vi "UHR-Fleezers Control (host) - Lorentz v4.vi"() -> ()   [LabVIEW 2014] (continued)
            n1313 = Subtract(x=w2088, y=w2087) -> (x-y=w2092:dbl)
            n1314 = local write "BD 1 Frequency 2 (MHz)"(w2071) -> ()
            n1315 = Subtract(x=w2082, y=w2071) -> (x-y=w2093:dbl)
            n1316 = Square(x=w2092) -> (x^2=w2090:dbl)
            n1317 = Square(x=w2093) -> (x^2=w2091:dbl)
            n1318 = Add(x=w2091, y=w2090) -> (x+y=w2089:dbl)
            n1319 = Square Root(x=w2089) -> (sqrt(x)=w2086:dbl)
            n1320 = property on="Initial delta (MHz)" class="DigNum (strict)"("Val(Sgnl)"=w2086) -> ()  [unwired: 2 in, 2 out]
            n1321 = local write "Trap Delta (MHz)"(w2086) -> ()
          }
          frame True {
          }
        }
      }
      event "manual raster set": Value Change {
        n1322 = event-data() -> ()  [unwired: 7 out]
        n1323 = flat-sequence {
          frame #0 {
            n1324 = Replace Array Subset(array=u32[] [0] ("Index Values"), new element="manual raster set", index=0) -> (w2113:u32[])
            n1325 = property on="Saved AOD Raster Scan Parameter Sets" class="Arr (strict)"("Index Values"=w2113) -> ()  [unwired: 2 in, 2 out]
          }
          frame #1 {
            n1326 = property on="Load parameters" class="Bool (strict)"("Val(Sgnl)"=TRUE ("Value (Signaling)")) -> ()  [unwired: 2 in, 2 out]
          }
        }
      }
      event "Round T1 X": Value Change {
        n1327 = event-data() -> ()  [unwired: 7 out]
        n1328 = local read "BD 1 Frequency 1 (MHz)"() -> (w2120:dbl)
        n1329 = Round To Nearest(number=w2120) -> (nearest integer value=w2119:dbl)
        n1330 = property on="BD 1 Frequency 1 (MHz)" class="DigNum (strict)"("Val(Sgnl)"=w2119) -> ()  [unwired: 2 in, 2 out]
      }
      event "Round T2 X": Value Change {
        n1331 = event-data() -> ()  [unwired: 7 out]
        n1332 = local read "BD 1 Frequency 2 (MHz)"() -> (w2122:dbl)
        n1333 = Round To Nearest(number=w2122) -> (nearest integer value=w2121:dbl)
        n1334 = property on="BD 1 Frequency 2 (MHz)" class="DigNum (strict)"("Val(Sgnl)"=w2121) -> ()  [unwired: 2 in, 2 out]
      }
      event "Stop All": Value Change {
        n1335 = event-data() -> ()  [unwired: 7 out]
        n1336 = flat-sequence {
          tunnel: [w2128] -> w2126
          tunnel: [w2131] -> w2124
          tunnel: w2126 -> [w2131]
          tunnel: [TRUE] -> w2125
          frame #0 {
            n1337 = local read "Visa resource for valves"() -> (w2127:refnum<visa-resource-name>)
            n1338 = call "hamilton_controller.vi"("VISA resource name in"=w2127, "action"=T53."DISCONNECT") -> ("error out"=w2128:errorcluster)  [unwired: 8 in, 1 out]
          }
          frame #1 {
          }
        }
      }
      event "Delayed Interlace Start": Value Change {
        n1339 = event-data() -> ()  [unwired: 7 out]
        n1340 = flat-sequence {
          frame #0 {
            n1341 = Multiply(x="Delay to Interlace (s)", y=1000.0) -> (x*y=w2133:dbl)
            n1342 = Wait (ms)(milliseconds to wait=w2133) -> ()  [unwired: 1 out]
          }
          frame #1 {
            n1343 = property on="Laser interlacing mode" class="RadioBtnsControl (strict)"("Val(Sgnl)"=enum32{"Laser ON", "Laser OFF", "Interlace"}."Interlace" ("Value (Signaling)")) -> ()  [unwired: 2 in, 2 out]
          }
        }
      }
      event "BD 1 Amplitude 1 (%)", "BD 1 Amplitude 2 (%)", "BD 1 Amplitude 3 (%)", "BD 2 Amplitude 1 (%)", "BD 2 Amplitude 2 (%)", "BD 2 Amplitude 3 (%)", "Trap 1 ON", "Trap 2 ON", "Trap 3 ON", "Feedback On/Off", "All FB On/Off": Value Change {
        w2158 = i16 1 ("f")
        n1344 = event-data() -> ()  [unwired: 7 out]
        n1345 = local write "Trap 1 (ON/OFF)"("Trap 1 ON") -> ()
        n1346 = local write "Trap 2 (ON/OFF)"("Trap 2 ON") -> ()
        n1347 = Boolean To (0,1)(Boolean="Trap 3 ON") -> (0, 1=w2159:i16)
        n1348 = Boolean To (0,1)(Boolean="Trap 1 ON") -> (0, 1=w2160:i16)
        n1349 = Boolean To (0,1)(Boolean="Trap 2 ON") -> (0, 1=w2161:i16)
        n1350 = Select(t=w2161, s="Trap ON/OFF X or Y Amp?", f=w2158) -> (s? t:f=w2156:i16)
        n1351 = Select(t=w2160, s="Trap ON/OFF X or Y Amp?", f=w2158) -> (s? t:f=w2157:i16)
        n1352 = Select(t=w2159, s="Trap ON/OFF X or Y Amp?", f=w2158) -> (s? t:f=w2155:i16)
        n1353 = Select(t=w2158, s="Trap ON/OFF X or Y Amp?", f=w2161) -> (s? t:f=w2153:i16)
        n1354 = Select(t=w2158, s="Trap ON/OFF X or Y Amp?", f=w2160) -> (s? t:f=w2154:i16)
        n1355 = Select(t=w2158, s="Trap ON/OFF X or Y Amp?", f=w2159) -> (s? t:f=w2152:i16)
        n1356 = And(x="All FB On/Off", y="Feedback On/Off") -> (x .and. y?=w2150:cluster{"Set 1":bool, "Set 2":bool})
        n1357 = local read "BD 1 Amplitude 1 (%)"() -> (w2168:dbl)
        n1358 = local read "BD 1 Amplitude 2 (%)"() -> (w2167:dbl)
        n1359 = local read "BD 1 Amplitude 3 (%)"() -> (w2166:dbl)
        n1360 = Unbundle By Name(w2150) -> ("Set 1"=w2145:bool, "Set 2"=w2142:bool)
        n1361 = local read "Y RF Amplitude Limits (%)"() -> (w2138:T24)
        n1362 = local read "X RF Amplitude Limits (%)"() -> (w2139:T24)
        n1363 = local read "BD 2 Amplitude 1 (%)"() -> (w2169:dbl)
        n1364 = local read "BD 2 Amplitude 2 (%)"() -> (w2170:dbl)
        n1365 = local read "BD 2 Amplitude 3 (%)"() -> (w2171:dbl)
        n1366 = And(x="Trap 2 ON", y=w2142) -> (x .and. y?=w2140:bool)
        n1367 = And(x="Trap 1 ON", y=w2145) -> (x .and. y?=w2143:bool)
        n1368 = Multiply(x=w2157, y=w2168) -> (x*y=w2165:dbl)
        n1369 = Multiply(x=w2167, y=w2156) -> (x*y=w2163:dbl)
        n1370 = Multiply(x=w2166, y=w2155) -> (x*y=w2164:dbl)
        n1371 = Multiply(x=w2169, y=w2154) -> (x*y=w2172:dbl)
        n1372 = Multiply(x=w2170, y=w2153) -> (x*y=w2173:dbl)
        n1373 = Multiply(x=w2171, y=w2152) -> (x*y=w2174:dbl)
        n1374 = call "set RF board amplitude - interlace.vi"("Board 2 Amplitude Limits"=w2138, "Board 1 Amplitude Limits"=w2139, "FPGA VI Reference In"=w2137, "Board 2 Amplitude 3 (%)"=w2174, "Board 1 Amplitude 3 (%)"=w2164, "Board 2 Amplitude 2 (%)"=w2173, "Board 2 Amplitude 1 (%)"=w2172, "Board 1 Amplitude 2 (%)"=w2163, "Board 1 Amplitude 1 (%)"=w2165) -> ("error out"=w2147:errorcluster, "FPGA VI Reference Out"=w2148:T50)  [unwired: 1 in]
        n1375 = xnode "Read/Write Control"("FPGA VI Reference In"=w2148, "error in"=w2147, "FB On/Off Set 1"=w2143, "FB On/Off Set 2"=w2140) -> ("error out"=w2146:errorcluster)  [unwired: 1 out]
      }
      event "Load parameters": Value Change {
        n1376 = event-data() -> ()  [unwired: 7 out]
        n1377 = property on="Saved AOD Raster Scan Parameter Sets" class="Arr (strict)"() -> ("Index Values"=w2185:u32[])  [unwired: 2 in, 2 out]
        n1378 = Index Array(array=w2185, index=0) -> (element=w2182:u32)
        n1379 = local write "Load parameters"(FALSE ("Load parameters")) -> ()
        n1380 = Index Array(array="Saved AOD Raster Scan Parameter Sets", index=w2182) -> (element=w2181:T55)
        n1381 = Unbundle By Name(w2181) -> ("Scan Range AOD (nm) 2"=w2180:dbl, "Step Size AOD (nm) 2"=w2179:dbl, "Scan Speed AOD (nm/s) 2"=w2178:dbl, "Number of scans (AOD) 2"=w2177:u16)
        n1382 = flat-sequence {
          tunnel: w2180 -> [w2188]
          tunnel: w2179 -> [w2187]
          tunnel: w2178 -> [w2186]
          tunnel: w2177 -> [w2189]
          frame #0 {
            n1383 = local write "Scan Speed (nm/s)"(w2186) -> ()
            n1384 = local write "Scan Range (nm)"(w2188) -> ()
            n1385 = local write "Step Size (nm)"(w2187) -> ()
          }
          frame #1 {
            n1386 = property on="Number of F/B Scans (AOD)" class="DigNum (strict)"("Val(Sgnl)"=w2189) -> ()  [unwired: 2 in, 2 out]
          }
        }
      }
      event "Trap 1 (ON/OFF)", "Trap 2 (ON/OFF)": Value Change {
        n1387 = event-data() -> ()  [unwired: 7 out]
        n1388 = flat-sequence {
          tunnel: [w2199] -> w2194
          tunnel: w2194 -> [w2214]
          tunnel: [w2200] -> w2190
          frame #0 {
            n1389 = local read "Trap 1 ON"() -> (w2199:bool)
          }
          frame #1 {
            n1390 = Exclusive Or(1:w2214, 2:"Trap 1 (ON/OFF)") -> (0:w2207:bool)
            n1391 = Select(t="on", s="Trap 2 (ON/OFF)", f="off") -> (s? t:f=w2206:string)
            n1392 = Select(t="on", s="Trap 1 (ON/OFF)", f="off") -> (s? t:f=w2202:string)
            n1393 = Build Array("trap 1 ", w2202) -> (w2201:string[])
            n1394 = Build Array("trap 2 " ("f"), w2206) -> (w2204:string[])
            n1395 = Select(t=w2201, s=w2207, f=w2204) -> (s? t:f=w2200:string[])
            n1396 = property on="Trap 1 ON" class="Bool (strict)"("Val(Sgnl)"="Trap 1 (ON/OFF)") -> ()  [unwired: 2 in, 2 out]
            n1397 = property on="Trap 2 ON" class="Bool (strict)"("Val(Sgnl)"="Trap 2 (ON/OFF)") -> ()  [unwired: 2 in, 2 out]
          }
        }
        n1398 = local read "Saving..."() -> (w2193:bool)
        n1399 = local read "Save Event Log?"() -> (w2192:bool)
        n1400 = And(x=w2193, y=w2192) -> (x .and. y?=w2191:bool)
        n1401 = case shown="True" w2191 {
          tunnel: w2190 -> [_ w2198]
          frame False {
          }
          frame True {
            n1402 = local read "Time (s)"() -> (w2195:dbl)
            n1403 = local read "log file ref"() -> (w2197:refnum<file>)
            n1404 = Concatenate Strings(w2198) -> (w2196:string)
            n1405 = call "write to event log.vi"("log file ref"=w2197, "time"=w2195, "input string"=w2196) -> ()  [unwired: 8 in]
          }
        }
      }
      event "DIO count 1 (ticks)", "DIO count 2 (ticks)", "DIO count 3 (ticks)", "Interlace", "Number Interlace Sets", "Not-Interlacing Set", "BD 1 Delay (ticks)", "BD 2 Delay (Ticks)", "Next trap write delay (ticks)", "XY phase ext loop method", "Amp switch delay 2", "BD 2 Delay (Ticks) 2", "BD 1 Delay (ticks) 2": Value Change {
        n1406 = event-data() -> ()  [unwired: 7 out]
        n1407 = To Unsigned Byte Integer(number="Not-Interlacing Set") -> (unsigned 8bit integer=w2215:u8)
        n1408 = Add(x=u8 1 ("y"), y=w2215) -> (x+y=w2224:u8)
        n1409 = local read "DIO count 1 (ticks)"() -> (w2231:u16)
        n1410 = local read "DIO count 2 (ticks)"() -> (w2230:u16)
        n1411 = local read "DIO count 3 (ticks)"() -> (w2229:u16)
        n1412 = xnode "Read/Write Control"("FPGA VI Reference In"=w2217, "DIO count 1 (ticks)"=w2231, "DIO count 2 (ticks)"=w2230, "DIO count 3 (ticks)"=w2229, "Interlace ON/OFF"="Interlace", "Number Interlace Cycles"="Number Interlace Sets", "Interlace Off Parameters"=w2224, "BD 1 Delay (ticks)"="BD 1 Delay (ticks)", "BD 2 Delay (Ticks)"="BD 2 Delay (Ticks)", "Next trap write delay (ticks)"="Next trap write delay (ticks)") -> ("error out"=w2233:errorcluster)  [unwired: 1 in, 1 out]
        n1413 = Build Array(w2231, w2230, w2229) -> (w2223:u16[])
        n1414 = Split 1D Array(array=w2223, index="Number Interlace Sets") -> (first subarray=w2232:u16[])  [unwired: 1 out]
        n1415 = Index Array(array=w2223, index=w2215) -> (element=w2222:u16)
        n1416 = Add Array Elements(numeric array=w2232) -> (sum=w2226:u16)
        n1417 = Select(t=w2226, s="Interlace", f=w2222) -> (s? t:f=→"Total Counts (ticks)":u16)
      }
      event "Reset Feedback": Value Change {
        n1418 = event-data() -> ()  [unwired: 7 out]
        n1419 = Unbundle By Name("Reset Feedback") -> ("Set 1"=w2237:bool, "Set 2"=w2236:bool)
        n1420 = xnode "Read/Write Control"("FPGA VI Reference In"=w2234, "FB Reset Set 1"=w2237, "FB Reset Set 2"=w2236) -> ("error out"=w2235:errorcluster)  [unwired: 1 in, 1 out]
      }
      event "Trap intensity output range", "Trap Intensity PID Gains": Value Change {
        n1421 = event-data() -> ()  [unwired: 7 out]
        n1422 = xnode "Read/Write Control"("FPGA VI Reference In"=w2241, "FB Gains"="Trap Intensity PID Gains", "FB output range"="Trap intensity output range") -> ("error out"=w2242:errorcluster)  [unwired: 1 in, 1 out]
      }
      event "AI2 to Setpoint", "Setpoints (V)": Value Change {
        n1423 = event-data() -> ()  [unwired: 7 out]
        n1424 = xnode "Read/Write Control"("FPGA VI Reference In"=w2243) -> ("FPGA VI Reference Out"=w2246:T50, "error out"=w2245:errorcluster, "AI2 Y Sum Set 1"=w2253:i16, "AI2 Y Sum Set 2"=w2252:i16)  [unwired: 1 in]
        n1425 = Cluster To Array(cluster="AI2 to Setpoint") -> (array=w2256:bool[])
        n1426 = local read "AI2 (V)"() -> (w2254:cluster{"Set 1":dbl, "Set 2":dbl})
        n1427 = Or Array Elements(Boolean array=w2256) -> (logical OR=w2257:bool)
        n1428 = Bundle By Name(cluster=w2254, "Set 1"=w2253, "Set 2"=w2252) -> (w2251:cluster{"Set 1":dbl, "Set 2":dbl})
        n1429 = Divide(x=w2251, y=3276.7) -> (x/y=w2250:cluster{"Set 1":dbl, "Set 2":dbl})
        "AI2 (V)" <- w2250
        n1430 = case shown="True" w2257 {
          tunnel: [w2260 w2277] -> w2249
          tunnel: "AI2 to Setpoint" -> [_ w2273]
          tunnel: "Setpoints (V)" -> [w2261 w2276]
          tunnel: w2250 -> [_ w2270]
          frame False {
            n1431 = Multiply(x=3276.7, y=w2261) -> (x*y=w2262:cluster{"Set 1":dbl, "Set 2":dbl})
            n1432 = To Word Integer(number=w2262) -> (16bit integer=w2260:cluster{"Set 1":i16, "Set 2":i16})
          }
          frame True {
            n1433 = Unbundle By Name(w2270) -> ("Set 1"=w2269:dbl, "Set 2"=w2268:dbl)
            n1434 = Unbundle By Name(w2276) -> ("Set 1"=w2275:dbl, "Set 2"=w2274:dbl)
            n1435 = Unbundle By Name(w2273) -> ("Set 1"=w2272:bool, "Set 2"=w2271:bool)
            n1436 = Select(t=w2269, s=w2272, f=w2275) -> (s? t:f=w2267:dbl)
            n1437 = Select(t=w2268, s=w2271, f=w2274) -> (s? t:f=w2266:dbl)
            n1438 = Bundle By Name(cluster=w2276, "Set 1"=w2267, "Set 2"=w2266) -> (w2264:cluster{"Set 1":dbl, "Set 2":dbl})
            n1439 = local write "Setpoints (V)"(w2264) -> ()
            n1440 = Multiply(x=3276.7, y=w2264) -> (x*y=w2265:cluster{"Set 1":dbl, "Set 2":dbl})
            n1441 = To Word Integer(number=w2265) -> (16bit integer=w2277:cluster{"Set 1":i16, "Set 2":i16})
          }
        }
        n1442 = Unbundle By Name(w2249) -> ("Set 1"=w2248:i16, "Set 2"=w2247:i16)
        n1443 = xnode "Read/Write Control"("FPGA VI Reference In"=w2246, "error in"=w2245, "FB Setpoint Set 1"=w2248, "FB Setpoint Set 2"=w2247) -> ("error out"=w2244:errorcluster)  [unwired: 1 out]
      }
      event "+ phase (GI)", "- phase (GI)", "+ phase (GI) 2", "- phase (GI) 2", "+ phase (RI)", "- phase (RI)", "+ phase (Green FB)", "- phase (Green FB)", "- phase (BI AO)", "+ phase (BI AO)", "- phase (BI DO)", "+ phase (BI DO)": Value Change {
        n1444 = event-data() -> ()  [unwired: 7 out]
        n1445 = Or(x="+ phase (GI)", y="- phase (GI)") -> (x .or. y?=w2313:bool)
        n1446 = Negate(x="Phase adj. (GI)") -> (-x=w2318:i16)
        n1447 = Select(t=w2318, s="+ phase (GI)", f="Phase adj. (GI)") -> (s? t:f=w2317:i16)
        n1448 = Or(x="+ phase (GI) 2", y="- phase (GI) 2") -> (x .or. y?=w2304:bool)
        n1449 = Negate(x="Phase adj. (GI) 2") -> (-x=w2309:i16)
        n1450 = Select(t=w2309, s="+ phase (GI) 2", f="Phase adj. (GI) 2") -> (s? t:f=w2305:i16)
        n1451 = Negate(x="Phase adj. (RI)") -> (-x=w2303:i16)
        n1452 = Or(x="+ phase (RI)", y="- phase (RI)") -> (x .or. y?=w2299:bool)
        n1453 = Select(t=w2303, s="+ phase (RI)", f="Phase adj. (RI)") -> (s? t:f=w2298:i16)
        n1454 = Or(x="+ phase (Green FB)", y="- phase (Green FB)") -> (x .or. y?=w2292:bool)
        n1455 = Negate(x="Phase adj. (Green FB)") -> (-x=w2297:i16)
        n1456 = Select(t=w2297, s="+ phase (Green FB)", f="Phase adj. (Green FB)") -> (s? t:f=w2293:i16)
        n1457 = Negate(x="Phase adj. (BI AO)") -> (-x=w2291:i16)
        n1458 = Or(x="+ phase (BI AO)", y="- phase (BI AO)") -> (x .or. y?=w2281:bool)
        n1459 = Select(t=w2291, s="+ phase (BI AO)", f="Phase adj. (BI AO)") -> (s? t:f=w2283:i16)
        n1460 = Negate(x="Phase adj. (BI DO)") -> (-x=w2287:i16)
        n1461 = Or(x="+ phase (BI DO)", y="- phase (BI DO)") -> (x .or. y?=w2280:bool)
        n1462 = Select(t=w2287, s="+ phase (BI DO)", f="Phase adj. (BI DO)") -> (s? t:f=w2282:i16)
        n1463 = xnode "Read/Write Control"("FPGA VI Reference In"=w2279, "Phase count adjustment (GI)"=w2317, "Phase count adjustment (GI) 2"=w2305, "Phase count adjustment (RI)"=w2298, "Phase count adjustment (Green FB)"=w2293, "Phase count adjustment (BI AO)"=w2283, "Phase count adjustment (BI D)"=w2282) -> ("FPGA VI Reference Out"=w2315:T50, "error out"=w2316:errorcluster)  [unwired: 1 in]
        n1464 = xnode "Read/Write Control"("FPGA VI Reference In"=w2315, "error in"=w2316, "+ phase (GI)"=w2313, "+ phase (GI) 2"=w2304, "+ phase (RI)"=w2299, "+ phase (Green FB)"=w2292, "+ phase (BI AO)"=w2281, "+ phase (BI D)"=w2280) -> ("error out"=w2314:errorcluster)  [unwired: 1 out]
      }
      event "Green Laser ON/OFF", "Red Laser ON/OFF", "Blue Laser ON/OFF": Value Change {
        # "This loop shouldn't be initialized.  The main 'laser ON' settings should dominate and set the others."
        n1465 = event-data() -> ()  [unwired: 7 out]
        n1466 = property on="Red Laser ON" class="Bool (strict)"("Val(Sgnl)"="Red Laser ON/OFF") -> ()  [unwired: 2 in, 2 out]
        n1467 = property on="Blue Laser ON" class="Bool (strict)"("Val(Sgnl)"="Blue Laser ON/OFF") -> ()  [unwired: 2 in, 2 out]
        n1468 = property on="Green Laser ON" class="Bool (strict)"("Val(Sgnl)"="Green Laser ON/OFF") -> ()  [unwired: 2 in, 2 out]
      }
      event "Laser interlacing mode", "Green Laser ON", "Red Laser ON", "Blue Laser ON": Value Change {
        n1469 = event-data() -> ()  [unwired: 7 out]
        n1470 = local write "Green Laser ON/OFF"("Green Laser ON") -> ()
        n1471 = local write "Blue Laser ON/OFF"("Blue Laser ON") -> ()
        n1472 = local write "Red Laser ON/OFF"("Red Laser ON") -> ()
        n1473 = case shown="False" "Green Laser ON" {
          tunnel: "Laser interlacing mode" -> [_ w2379]
          tunnel: [enum32{"Laser ON", "Laser OFF", "Interlace"}."Laser OFF" ("Green laser mode") w2379] -> w2355
          tunnel: [FALSE w2375] -> w2354
          frame False {
          }
          frame True {
            n1474 = local read "Green FB On/Off"() -> (w2376:bool)
            n1475 = Equal?(x=w2379, y=enum32{"Laser ON", "Laser OFF", "Interlace"}."Interlace") -> (x = y?=w2377:bool)
            n1476 = And(x=w2377, y=w2376) -> (x .and. y?=w2375:bool)
          }
        }
        n1477 = case shown="True" "Red Laser ON" {
          tunnel: "Laser interlacing mode" -> [_ w2372]
          tunnel: [enum32{"Laser ON", "Laser OFF", "Interlace"}."Laser OFF" ("Green laser mode") w2372] -> w2351
          tunnel: [FALSE w2368] -> w2350
          frame False {
          }
          frame True {
            n1478 = local read "Red FB On/Off"() -> (w2369:bool)
            n1479 = Equal?(x=w2372, y=enum32{"Laser ON", "Laser OFF", "Interlace"}."Interlace") -> (x = y?=w2370:bool)
            n1480 = And(x=w2370, y=w2369) -> (x .and. y?=w2368:bool)
          }
        }
        n1481 = case shown="True" "Blue Laser ON" {
          tunnel: "Laser interlacing mode" -> [_ w2363]
          tunnel: [enum32{"Laser ON", "Laser OFF", "Interlace"}."Laser OFF" ("Green laser mode") w2363] -> w2347
          tunnel: [FALSE w2361] -> w2346
          frame False {
          }
          frame True {
            n1482 = local read "Blue FB On/Off"() -> (w2362:bool)
            n1483 = Equal?(x=w2363, y=enum32{"Laser ON", "Laser OFF", "Interlace"}."Interlace") -> (x = y?=w2364:bool)
            n1484 = And(x=w2364, y=w2362) -> (x .and. y?=w2361:bool)
          }
        }
        n1485 = xnode "Read/Write Control"("FPGA VI Reference In"=w2345, "Operating Mode"=w2355, "Operating Mode 2"=w2355, "Green FB On/Off"=w2354, "Red Laser Operating Mode"=w2351, "RI Operating Mode 2"=w2351, "Red FB On/Off"=w2350, "BI Operating Mode (AO)"=w2347, "Blue Laser Operating Mode (D)"=w2347, "Blue FB On/Off"=w2346) -> ("error out"=w2356:errorcluster)  [unwired: 1 in, 1 out]
        n1486 = local read "Red FB On/Off"() -> (w2328:bool)
        n1487 = local read "Green FB On/Off"() -> (w2330:bool)
        n1488 = local read "Green Laser ON"() -> (w2329:bool)
        n1489 = local read "Red Laser ON"() -> (w2327:bool)
        n1490 = And(x=w2328, y=w2327) -> (x .and. y?=w2333:bool)
        n1491 = And(x=w2330, y=w2329) -> (x .and. y?=w2339:bool)
        n1492 = local read "Red laser intensity (V)"() -> (w2332:dbl)
        n1493 = local read "Red FB Setpoint (mV)"() -> (w2331:dbl)
        n1494 = local read "Green FB Setpoint (mV)"() -> (w2342:dbl)
        n1495 = local read "Green laser intensity (V)"() -> (w2344:dbl)
        n1496 = Multiply(x=w2332, y=1000.0) -> (x*y=w2336:dbl)
        n1497 = Subtract(x=w2331, y=5.0) -> (x-y=w2335:dbl)
        n1498 = Multiply(x=w2344, y=1000.0) -> (x*y=w2341:dbl)
        n1499 = Subtract(x=w2342, y=5.0) -> (x-y=w2340:dbl)
        n1500 = Less Or Equal?(x=w2336, y=w2335) -> (x <= y?=w2334:bool)
        n1501 = Less Or Equal?(x=w2341, y=w2340) -> (x <= y?=w2338:bool)
        n1502 = And(x=w2333, y=w2334) -> (x .and. y?=w2323:bool)
        n1503 = And(x=w2339, y=w2338) -> (x .and. y?=w2324:bool)
        n1504 = Or(x=w2324, y=w2323) -> (x .or. y?=w2322:bool)
        n1505 = case shown="True" w2322 {
          frame False {
            n1506 = local write "Laser Intensity Low (bugs to fix)"(FALSE ("Laser Intensity Low")) -> ()
          }
          frame True {
            n1507 = local write "Laser Intensity Low (bugs to fix)"(TRUE ("Laser Intensity Low")) -> ()
          }
        }
      }
      event "Invert laser interlacing": Value Change {
        n1508 = event-data() -> ()  [unwired: 7 out]
        n1509 = xnode "Read/Write Control"("FPGA VI Reference In"=w2380, "Invert GI"="Invert laser interlacing", "Invert GI 2"="Invert laser interlacing", "Invert RI"="Invert laser interlacing", "Invert RI 2"="Invert laser interlacing", "Invert BI (AO)"="Invert laser interlacing", "Invert BI (D)"="Invert laser interlacing") -> ("error out"=w2382:errorcluster)  [unwired: 1 in, 1 out]
      }
      event "Green FB Setpoint (mV)", "Green FB Gains", "Green FB On/Off", "Green Intensity % (FB OFF)", "Green int current ON count adj": Value Change {
        n1510 = event-data() -> ()  [unwired: 7 out]
        n1511 = local read "Green FB Setpoint (mV)"() -> (w2402:dbl)
        n1512 = Multiply(x=w2402, y=3.2767) -> (x*y=w2401:dbl)
        n1513 = local read "Green Intensity % (FB OFF)"() -> (w2405:dbl)
        n1514 = Multiply(x=w2405, y=655.35) -> (x*y=w2406:dbl)
        n1515 = To Unsigned Word Integer(number=w2406) -> (unsigned 16bit integer=w2404:u16)
        n1516 = local read "Green int current ON count adj"() -> (w2408:u32)
        n1517 = local read "Laser interlacing mode"() -> (w2399:enum32{"Laser ON", "Laser OFF", "Interlace"})
        n1518 = local read "Green FB Gains"() -> (w2396:T14)
        n1519 = local read "Green Laser ON"() -> (w2400:bool)
        n1520 = local read "Green FB On/Off"() -> (w2409:bool)
        n1521 = Equal?(x=w2399, y=enum32{"Laser ON", "Laser OFF", "Interlace"}."Interlace") -> (x = y?=w2397:bool)
        n1522 = Unbundle By Name(w2396) -> ("proportional gain (Kc)"=w2395:i16, "integral gain (Kc*Ts/Ti)"=w2394:i16, "derivative gain (Kc*Td/Ts)"=w2393:i16)
        n1523 = Compound Arithmetic op=AND(w2397, w2409, w2400) -> (w2383:bool)
        n1524 = local read "Green FB Setpoint (mV)"() -> (w2387:dbl)
        n1525 = local read "Green laser intensity (V)"() -> (w2390:dbl)
        n1526 = xnode "Read/Write Control"("FPGA VI Reference In"=w2392, "Green FB Setpoint"=w2401, "Green FB On/Off"=w2383, "Current Out"=w2404, "Green int current ON count adj"=w2408, "P3"=w2395, "I3"=w2394, "D3"=w2393) -> ("error out"=w2410:errorcluster)  [unwired: 1 in, 1 out]
        n1527 = Multiply(x=w2390, y=1000.0) -> (x*y=w2386:dbl)
        n1528 = Subtract(x=w2387, y=5.0) -> (x-y=w2385:dbl)
        n1529 = Less Or Equal?(x=w2386, y=w2385) -> (x <= y?=w2384:bool)
        n1530 = And(x=w2383, y=w2384) -> (x .and. y?=w2391:bool)
        n1531 = case shown="True" w2391 {
          frame False {
            n1532 = local write "Laser Intensity Low (bugs to fix)"(FALSE ("Laser Intensity Low")) -> ()
          }
          frame True {
            n1533 = local write "Laser Intensity Low (bugs to fix)"(TRUE ("Laser Intensity Low")) -> ()
          }
        }
      }
      event "Blue FB Setpoint (mV)", "Blue FB Gains", "Blue FB On/Off", "Blue Intensity % (FB OFF)", "Blue int AO ON count adjust": Value Change {
        # "Triggers blue laser serial command"
        # "16 bit analog out"
        n1534 = event-data() -> ()  [unwired: 7 out]
        n1535 = Multiply(x="Blue FB Setpoint (mV)", y=3.2767) -> (x*y=w2430:dbl)
        n1536 = Multiply(x="Blue Intensity % (FB OFF)", y=0.8) -> (x*y=w2413:dbl)
        n1537 = Number To Decimal String(number=w2413) -> (decimal integer string=w2414:string)  [unwired: 1 in]
        n1538 = Multiply(x="Blue Intensity % (FB OFF)", y=655.35) -> (x*y=w2433:dbl)
        n1539 = local write "Blue Laser Power (mW)\n(Constant Power Mode)"(w2414) -> ()
        n1540 = To Unsigned Word Integer(number=w2433) -> (unsigned 16bit integer=w2432:u16)
        n1541 = local read "Laser interlacing mode"() -> (w2428:enum32{"Laser ON", "Laser OFF", "Interlace"})
        n1542 = Unbundle By Name("Blue FB Gains") -> ("proportional gain (Kc)"=w2425:i16, "integral gain (Kc*Ts/Ti)"=w2424:i16, "derivative gain (Kc*Td/Ts)"=w2423:i16)
        n1543 = local read "Blue Laser ON"() -> (w2418:bool)
        n1544 = Equal?(x=w2428, y=enum32{"Laser ON", "Laser OFF", "Interlace"}."Interlace") -> (x = y?=w2426:bool)
        n1545 = Compound Arithmetic op=AND(w2426, "Blue FB On/Off", w2418) -> (w2429:bool)
        n1546 = xnode "Read/Write Control"("FPGA VI Reference In"=w2417, "Blue FB Setpoint"=w2430, "Blue FB On/Off"=w2429, "BI Current Out"=w2432, "Blue current ON count adj (AO)"="Blue int AO ON count adjust", "P5"=w2425, "I5"=w2424, "D5"=w2423) -> ("error out"=w2435:errorcluster)  [unwired: 1 in, 1 out]
      }
      event "Red FB Setpoint (mV)", "Red FB Gains", "Red FB On/Off", "Red Intensity % (FB OFF)": Value Change {
        n1547 = event-data() -> ()  [unwired: 7 out]
        n1548 = local read "Red FB Setpoint (mV)"() -> (w2456:dbl)
        n1549 = Multiply(x=w2456, y=3.2767) -> (x*y=w2455:dbl)
        n1550 = local read "Red Intensity % (FB OFF)"() -> (w2446:dbl)
        n1551 = Multiply(x=w2446, y=655.35) -> (x*y=w2459:dbl)
        n1552 = To Unsigned Word Integer(number=w2459) -> (unsigned 16bit integer=w2458:u16)
        n1553 = local read "Laser interlacing mode"() -> (w2453:enum32{"Laser ON", "Laser OFF", "Interlace"})
        n1554 = local read "Red FB Gains"() -> (w2450:T14)
        n1555 = local read "Red Laser ON"() -> (w2454:bool)
        n1556 = local read "Red FB On/Off"() -> (w2461:bool)
        n1557 = Equal?(x=w2453, y=enum32{"Laser ON", "Laser OFF", "Interlace"}."Interlace") -> (x = y?=w2451:bool)
        n1558 = Unbundle By Name(w2450) -> ("proportional gain (Kc)"=w2449:i16, "integral gain (Kc*Ts/Ti)"=w2448:i16, "derivative gain (Kc*Td/Ts)"=w2447:i16)
        n1559 = Compound Arithmetic op=AND(w2451, w2461, w2454) -> (w2438:bool)
        n1560 = local read "Red laser intensity (V)"() -> (w2437:dbl)
        n1561 = local read "Red FB Setpoint (mV)"() -> (w2436:dbl)
        n1562 = xnode "Read/Write Control"("FPGA VI Reference In"=w2445, "Red FB Setpoint"=w2455, "Red FB On/Off"=w2438, "RI Current Out"=w2458, "P4"=w2449, "I4"=w2448, "D4"=w2447) -> ("error out"=w2462:errorcluster)  [unwired: 1 in, 1 out]
        n1563 = Multiply(x=w2437, y=1000.0) -> (x*y=w2442:dbl)
        n1564 = Subtract(x=w2436, y=5.0) -> (x-y=w2441:dbl)
        n1565 = Less Or Equal?(x=w2442, y=w2441) -> (x <= y?=w2440:bool)
        n1566 = And(x=w2438, y=w2440) -> (x .and. y?=w2439:bool)
        n1567 = case shown="False" w2439 {
          frame False {
            n1568 = local write "Laser Intensity Low (bugs to fix)"(FALSE ("Laser Intensity Low")) -> ()
          }
          frame True {
            n1569 = local write "Laser Intensity Low (bugs to fix)"(TRUE ("Laser Intensity Low")) -> ()
          }
        }
      }
      event "+ phase (APD 1 Gate)", "- phase (APD 1 Gate)", "+ phase (APD 2 Gate)", "- phase (APD 2 Gate)", "+ phase (APD 3 Gate)", "- phase (APD 3 Gate)", "+ phase (APD Acq)", "- phase (APD Acq)": Value Change {
        n1570 = event-data() -> ()  [unwired: 7 out]
        n1571 = local read "Phase Adj. (APD 1 Gate)"() -> (w2485:i16)
        n1572 = Or(x="- phase (APD 1 Gate)", y="+ phase (APD 1 Gate)") -> (x .or. y?=w2487:bool)
        n1573 = Negate(x=w2485) -> (-x=w2492:i16)
        n1574 = Select(t=w2492, s="+ phase (APD 1 Gate)", f=w2485) -> (s? t:f=w2491:i16)
        n1575 = local read "Phase Adj. (APD 2 Gate)"() -> (w2482:i16)
        n1576 = Or(x="- phase (APD 2 Gate)", y="+ phase (APD 2 Gate)") -> (x .or. y?=w2480:bool)
        n1577 = Negate(x=w2482) -> (-x=w2484:i16)
        n1578 = Select(t=w2484, s="+ phase (APD 2 Gate)", f=w2482) -> (s? t:f=w2481:i16)
        n1579 = Negate(x="Phase Adj. (APD 3 Gate)") -> (-x=w2479:i16)
        n1580 = Or(x="- phase (APD 3 Gate)", y="+ phase (APD 3 Gate)") -> (x .or. y?=w2475:bool)
        n1581 = Select(t=w2479, s="+ phase (APD 3 Gate)", f="Phase Adj. (APD 3 Gate)") -> (s? t:f=w2476:i16)
        n1582 = local read "Phase Adj. (APD Acq)"() -> (w2473:i16)
        n1583 = Or(x="- phase (APD Acq)", y="+ phase (APD Acq)") -> (x .or. y?=w2471:bool)
        n1584 = Negate(x=w2473) -> (-x=w2474:i16)
        n1585 = Select(t=w2474, s="+ phase (APD Acq)", f=w2473) -> (s? t:f=w2472:i16)
        n1586 = xnode "Read/Write Control"("FPGA VI Reference In"=w2465, "Phase count adjustment (APD 1 Gate)"=w2491, "Phase count adjustment (APD 2 Gate)"=w2481, "Phase count adjustment (APD 3 Gate)"=w2476, "Phase Count Adjustment (APD Acq)"=w2472) -> ("FPGA VI Reference Out"=w2489:T50, "error out"=w2490:errorcluster)  [unwired: 1 in]
        n1587 = xnode "Read/Write Control"("FPGA VI Reference In"=w2489, "error in"=w2490, "+ phase (APD 1 Gate)"=w2487, "+ phase (APD 2 Gate)"=w2480, "+ phase (APD 3 Gate)"=w2475, "+ phase (APD Acq)"=w2471) -> ("error out"=w2488:errorcluster)  [unwired: 1 out]
      }
      event "Invert APD Gate", "APD Gate ON Count", "APD Gate OFF Count", "APD Gate", "APD Integration Time (s)", "APD AO Scale Factor", "Duty Frequency (ON 1/N cycles)", "Interlace ON count", "Interlace OFF count": Value Change {
        n1588 = event-data() -> ()  [unwired: 7 out]
        n1589 = Add(x="Interlace ON count", y="Interlace OFF count") -> (x+y=w2499:u16)
        n1590 = Add(x="APD Gate ON Count", y="APD Gate OFF Count") -> (x+y=w2510:u16)
        n1591 = Multiply(x="Duty Frequency (ON 1/N cycles)", y=w2499) -> (x*y=w2495:u16)
        "Green AI Count" <- w2495
        "Red AI Count" <- w2495
        "Blue AI Count" <- w2495
        n1592 = Subtract(x=w2495, y="Interlace ON count") -> (x-y=w2498:u16)
        n1593 = Multiply(x=w2510, y="Duty Frequency (ON 1/N cycles)") -> (x*y=w2509:u16)
        n1594 = Subtract(x=w2509, y="APD Gate ON Count") -> (x-y=w2508:u16)
        n1595 = local read "DMA Update Period (s)"() -> (w2511:dbl)
        n1596 = Multiply(x="APD Integration Time (s)", y=40000000.0) -> (x*y=w2515:dbl)
        n1597 = Reciprocal(x="APD Integration Time (s)") -> (1/x=→"APD Acq Rate (Hz)":dbl)
        n1598 = To Unsigned Long Integer(number=w2515) -> (unsigned 32bit integer=w2501:u32)
        "APD Int. Count" <- w2501
        n1599 = local read "Number of APDs"() -> (w2494:u8)
        n1600 = Divide(x=w2511, y="APD Integration Time (s)") -> (x/y=w2513:dbl)
        n1601 = Multiply(x=w2494, y=w2513) -> (x*y=w2512:dbl)
        n1602 = local write "APD Samples/FIFO Acq."(w2513) -> ()
        n1603 = local write "APD Elements/DMA read"(w2512) -> ()
        n1604 = xnode "Read/Write Control"("FPGA VI Reference In"=w2493, "Invert APD Gate"="Invert APD Gate", "APD Gate ON Count"="APD Gate ON Count", "APD Gate OFF Count"=w2508, "APD Acq Rate Count"=w2501, "APD Gate Operating Mode"="APD Gate", "APD AO scale factor"="APD AO Scale Factor", "Green interlace ON count"="Interlace ON count", "Green interlace OFF count"=w2498, "Green interlace ON count 2"="Interlace ON count", "Green interlace OFF count 2"=w2498, "Green FB Count"=w2495, "Red interlace ON count"="Interlace ON count", "Red interlace OFF count"="Interlace OFF count", "Blue ON count (AO)"="Interlace ON count", "Blue OFF count (AO)"="Interlace OFF count", "Blue interlace OFF count (D)"="Interlace OFF count", "Blue interlace ON count (D)"="Interlace ON count") -> ("error out"=w2517:errorcluster)  [unwired: 1 in, 1 out]
      }
      event "Neg. TTrig FPGA": Value Change {
        n1605 = event-data() -> ()  [unwired: 7 out]
        n1606 = xnode "Read/Write Control"("FPGA VI Reference In"=w2518, "TTrig Negate Pos"="Neg. TTrig FPGA") -> ()  [unwired: 1 in, 2 out]
      }
      event "Test ttrig": Value Change {
        n1607 = event-data() -> ()  [unwired: 7 out]
        n1608 = xnode "Read/Write Control"("FPGA VI Reference In"=w2520, "TTrig?"=TRUE) -> ("error out"=w2522:errorcluster)  [unwired: 1 in, 1 out]
      }
      event "Number of F/B Scans (AOD)", "Scan Speed (nm/s)", "Scan BD", "Initial delta (MHz)", "Step Size (nm)", "Scan Range (nm)": Value Change {
        w2586 = 123.0  # AOM cal (nm/MHz)
        n1609 = event-data() -> ()  [unwired: 7 out]
        n1610 = local read "BD 1 Frequency 1 (MHz)"() -> (w2569:dbl)
        n1611 = local read "AOM X Cal (nm/MHz)"() -> (w2561:dbl)
        n1612 = local read "X RF Frequency Limits (MHz)"() -> (w2573:T24)
        n1613 = local read "Y RF Frequency Limits (MHz)"() -> (w2570:T24)
        n1614 = local read "BD 2 Frequency 1 (MHz)"() -> (w2575:dbl)
        n1615 = Negate(x="Scan Range (nm)") -> (-x=w2539:dbl)
        n1616 = Divide(x=w2539, y=w2561) -> (x/y=w2543:dbl)
        n1617 = Select(t=w2573, s="Scan BD", f=w2570) -> (s? t:f=w2572:T24)
        n1618 = Select(t=w2569, s="Scan BD", f=w2575) -> (s? t:f=w2574:dbl)
        n1619 = Unbundle By Name(w2572) -> ("Maximum"=w2581:dbl, "Minimum"=w2580:dbl)
        n1620 = Add(x=w2543, y=w2574) -> (x+y=w2578:dbl)
        n1621 = Divide(x=w2539, y="Step Size (nm)") -> (x/y=w2558:dbl)
        n1622 = Divide(x="Step Size (nm)", y=w2561) -> (x/y=w2567:dbl)
        n1623 = Absolute Value(x=w2558) -> (abs(x)=w2542:dbl)
        n1624 = Sign(1:w2539) -> (0:w2540:dbl)
        n1625 = In Range and Coerce(upper limit=w2581, x=w2578, lower limit=w2580) -> (coerced(x)=w2577:dbl, In Range?=w2579:bool)
        n1626 = To Unsigned Quad Integer(1:w2542) -> (0:w2557:u64)
        "Scan steps (AOD)" <- w2557
        n1627 = call "IR AOM freq to word.vi"("Frequency In (MHz)"=w2567) -> ("Frequency Word Out (double)"=w2564:dbl)
        n1628 = Multiply(x=w2540, y=w2564) -> (x*y=w2541:dbl)
        n1629 = Subtract(x=w2578, y=w2577) -> (x-y=w2576:dbl)
        n1630 = To Quad Integer(1:w2541) -> (0:w2563:i64)
        "Incr. int (AOD)" <- w2563
        n1631 = Subtract(x=w2543, y=w2576) -> (x-y=w2562:dbl)
        "Scan Range (MHz)" <- w2562
        n1632 = Select(t=w2543, s=w2579, f=w2562) -> (s? t:f=w2582:dbl)
        n1633 = Multiply(x=w2562, y=w2561) -> (x*y=w2560:dbl)
        n1634 = Decrement(x=w2557) -> (x-1=w2610:u64)
        n1635 = Negate(x=w2560) -> (-x=w2556:dbl)
        n1636 = local write "Scan Range (nm)"(w2556) -> ()
        n1637 = Divide(x=w2582, y=w2610) -> (x/y=w2566:dbl)
        "Scan Increment (MHz)" <- w2566
        n1638 = call "IR AOM freq to word.vi"("Frequency In (MHz)"=w2566) -> ("Frequency Word Out (double)"=w2565:dbl)
        n1639 = Divide(x="Step Size (nm)", y="Scan Speed (nm/s)") -> (x/y=w2553:dbl)
        n1640 = To Quad Integer(1:w2565) -> ()  [unwired: 1 out]
        n1641 = local read "Number Interlace Sets"() -> (w2537:u8)
        n1642 = local read "AI Count (ticks)"() -> (w2538:u16)
        n1643 = local read "Total Counts (ticks)"() -> (w2536:u16)
        n1644 = local read "# Samples/trap"() -> (w2568:u32)
        n1645 = Multiply(x=w2538, y=w2537) -> (x*y=w2535:u16)
        n1646 = Divide(x=w2536, y=w2535) -> (x/y=w2534:dbl)
        n1647 = Select(t=w2569, s="Scan BD", f=w2575) -> (s? t:f=w2607:dbl)
        "Initial freq. (MHz)" <- w2607
        n1648 = Add(x=w2582, y=w2607) -> (x+y=→"Final freq. (MHz)":dbl)
        n1649 = Divide(x=w2536, y=40000000.0) -> (x/y=w2552:dbl)
        n1650 = Divide(x=w2553, y=w2552) -> (x/y=w2551:dbl)
        n1651 = To Unsigned Quad Integer(1:w2551) -> (0:w2526:u64)
        n1652 = Quotient & Remainder(x=w2526, y=u64 2) -> (x-y*floor(x/y)=w2530:u64)  [unwired: 1 out]
        n1653 = Equal?(x=w2530, y=u64 0) -> (x = y?=w2528:bool)
        n1654 = Decrement(x=w2526) -> (x-1=w2527:u64)
        n1655 = Select(t=w2526, s=w2528, f=w2527) -> (s? t:f=w2525:u64)
        "Cycles/step (AOD)" <- w2525
        n1656 = xnode "Read/Write Control"("FPGA VI Reference In"=w2524, "Scan steps"=w2557, "Number of scans"="Number of F/B Scans (AOD)", "Cycles per step"=w2525, "Scan freq.  increment"=w2563, "Scan BD"="Scan BD") -> ("error out"=w2616:errorcluster)  [unwired: 1 in, 1 out]
        n1657 = Multiply(x=w2557, y=w2525) -> (x*y=w2611:u64)
        n1658 = Multiply(x=w2611, y=u64 2) -> (x*y=w2533:u64)
        n1659 = Multiply(x=w2534, y=w2533) -> (x*y=w2532:dbl)
        "Data points/scan (f/b)" <- w2532
        n1660 = Multiply(x=w2532, y="Number of F/B Scans (AOD)") -> (x*y=w2614:dbl)
        "Data points/scans" <- w2614
        n1661 = Divide(x=w2614, y=w2568) -> (x/y=→"N sets should be saved":dbl)
        n1662 = Multiply(x=w2611, y=w2552) -> (x*y=w2550:dbl)
        "Time/Scan (s) (AOD)" <- w2550
        n1663 = Select(t=w2582, s="Scan BD", f=0.0) -> (s? t:f=w2608:dbl)
        n1664 = Select(t=0.0, s="Scan BD", f=w2582) -> (s? t:f=w2604:dbl)
        n1665 = local read "BD 2 Frequency 2 (MHz)"() -> (w2600:dbl)
        n1666 = local read "BD 1 Frequency 2 (MHz)"() -> (w2603:dbl)
        n1667 = Add(x=w2604, y=w2575) -> (x+y=w2601:dbl)
        n1668 = Add(x=w2569, y=w2608) -> (x+y=w2602:dbl)
        n1669 = Multiply(x=w2550, y=2.0) -> (x*y=w2549:dbl)
        n1670 = Multiply(x=w2549, y="Number of F/B Scans (AOD)") -> (x*y=w2546:dbl)
        n1671 = Divide(x=w2546, y=60.0) -> (x/y=→"Time to Finish All (min)":dbl)
        n1672 = Add(x="Trap 2 Bead Size (nm)", y="Trap 1 Bead Size (nm)") -> (x+y=w2590:dbl)
        n1673 = Divide(x=w2590, y=2.0) -> (x/y=w2584:dbl)
        n1674 = local read "Initial delta (MHz)"() -> (w2587:dbl)
        n1675 = Subtract(x=w2601, y=w2600) -> (x-y=w2598:dbl)
        n1676 = Subtract(x=w2602, y=w2603) -> (x-y=w2599:dbl)
        n1677 = Square(x=w2598) -> (x^2=w2597:dbl)
        n1678 = Square(x=w2599) -> (x^2=w2596:dbl)
        n1679 = Add(x=w2596, y=w2597) -> (x+y=w2595:dbl)
        n1680 = Square Root(x=w2595) -> (sqrt(x)=w2594:dbl)
        "Final delta (MHz)" <- w2594
        n1681 = Multiply(x=w2586, y=w2594) -> (x*y=w2593:dbl)
        n1682 = Multiply(x=w2587, y=w2586) -> (x*y=w2585:dbl)
        n1683 = Subtract(x=w2585, y=w2584) -> (x-y=→"Initial sep (nm)":dbl)
        n1684 = Subtract(x=w2593, y=w2584) -> (x-y=→"Final sep (nm)":dbl)
      }
      event "Freq or Amp switch first", "Swap F1 and F2", "Freq switch delay", "Amp switch delay": Value Change {
        n1685 = event-data() -> ()  [unwired: 7 out]
        n1686 = local read "Amp switch delay"() -> (w2618:u16)
        n1687 = local read "Swap F1 and F2"() -> (w2619:bool)
        n1688 = xnode "Read/Write Control"("FPGA VI Reference In"=w2617, "Swap F1 and F2"=w2619, "Amp switch delay"=w2618) -> ("error out"=w2620:errorcluster)  [unwired: 1 in, 1 out]
      }
      event "Scan steps (MCL)", "Number of scans (MCL)", "Scan Range (V)\n(of steps)", "2D or 1D Scan", "N APD Samp/step", "Fast Scan Dir", "Continuous MCL Scanning", "Scan lines (y)": Value Change {
        w2623 = 32767.0 ("y")
        n1689 = event-data() -> ()  [unwired: 7 out]
        n1690 = Select(t="Scan lines (y)", s="2D or 1D Scan", f="Number of scans (MCL)") -> (s? t:f=w2628:u64)
        n1691 = Decrement(x="Scan steps (MCL)") -> (x-1=w2644:u64)
        n1692 = Divide(x="Scan Range (V)\n(of steps)", y=w2644) -> (x/y=w2643:dbl)
        "Desired Scan Incr (V)" <- w2643
        n1693 = local read "APD Integration Time (s)"() -> (w2636:dbl)
        n1694 = Multiply(x=w2643, y=w2623) -> (x*y=w2652:dbl)
        n1695 = Divide(x=w2652, y=10.0) -> (x/y=w2642:dbl)
        "Desired incr (int)" <- w2642
        n1696 = local read "Update Count (MCL)"() -> (w2648:u32)
        n1697 = Round Toward -Infinity(1:w2642) -> (0:w2651:dbl)
        n1698 = To Word Integer(number=w2651) -> (16bit integer=w2626:i16)
        "Actual Incr. int (MCL)" <- w2626
        n1699 = Multiply(x=w2636, y=40000000.0) -> (x*y=w2649:dbl)
        n1700 = Divide(x=w2649, y=w2648) -> (x/y=w2647:dbl)
        n1701 = Multiply(x=i16 10, y=w2626) -> (x*y=w2624:i16)
        n1702 = Multiply(x="N APD Samp/step", y=w2647) -> (x*y=w2646:dbl)
        "Cycles/step (MCL)" <- w2646
        n1703 = Divide(x=w2624, y=w2623) -> (x/y=→"Actual MCL Inc (V)":dbl)
        n1704 = Multiply(x="N APD Samp/step", y="Scan steps (MCL)") -> (x*y=w2638:dbl)
        n1705 = local read "APD Samples/FIFO Acq."() -> (w2635:dbl)
        n1706 = Multiply(x=w2638, y=u64 2) -> (x*y=w2637:dbl)
        "Data points/scan (f+b)" <- w2637
        n1707 = Multiply(x=w2637, y=w2628) -> (x*y=w2655:dbl)
        "Data points/scans (MCL)" <- w2655
        n1708 = Multiply(x=w2636, y=w2637) -> (x*y=w2629:dbl)
        "Time/f+b scan (s) (MCL)" <- w2629
        n1709 = Divide(x=w2655, y=w2635) -> (x/y=→"N sets should be saved (MCL)":dbl)
        n1710 = Multiply(x=w2629, y=w2628) -> (x*y=→"Total Time (s)":dbl)
        n1711 = Not(x="Fast Scan Dir") -> (.not. x?=w2633:bool)
        n1712 = xnode "Read/Write Control"("FPGA VI Reference In"=w2621, "Scan steps (MCL)"="Scan steps (MCL)", "Number of scans (MCL)"=w2628, "Cycles per step (MCL)"=w2646, "Scan freq.  increment (MCL)"=w2626, "1D or 2D Scan?"="2D or 1D Scan", "MCL Scan Axis"=w2633, "Cont. Scan (MCL)"="Continuous MCL Scanning") -> ("error out"=w2657:errorcluster)  [unwired: 1 in, 1 out]
      }
      event "Read Cal": Value Change {
        w2696 = 1000.0 ("y")
        w2679 = T38."big-endian, network order" ("byte order (0:big-endian, network order)")
        w2680 = -1 ("count (1)")
        n1713 = event-data() -> ()  [unwired: 7 out]
        n1714 = local read "Save file name"() -> (w2712:path)
        n1715 = local write "Read Cal"(FALSE ("Read Cal")) -> ()
        n1716 = Strip Path(path=w2712) -> (stripped path=w2711:path)  [unwired: 1 out]
        n1717 = Path To String(path=w2711) -> (string=w2688:string)
        n1718 = Concatenate Strings(w2688, "\\current.cal" ("string")) -> (w2709:string)
        n1719 = Concatenate Strings(w2688, "\\current.off" ("string")) -> (w2686:string)
        n1720 = String To Path(string=w2709) -> (path=w2708:path)
        n1721 = String To Path(string=w2686) -> (path=w2683:path)
        n1722 = Open/Create/Replace File(file path (use dialog)=w2708, operation (0:open)=T39."open", access (0:read/write)=enum16{"read/write", "read-only", "write-only"}."read-only") -> (refnum out=w2715:refnum<file>, error out=w2704:errorcluster)  [unwired: 1 in, 3 out]
        n1723 = Open/Create/Replace File(file path (use dialog)=w2683, operation (0:open)=T39."open", access (0:read/write)=enum16{"read/write", "read-only", "write-only"}."read-only") -> (refnum out=w2682:refnum<file>)  [unwired: 1 in, 4 out]
        n1724 = Deny Access(4:w2704, 7:w2715) -> (0:w2703:errorcluster, 3:w2707:refnum<file>)  [unwired: 1 out]
        n1725 = Deny Access(7:w2682) -> (3:w2681:refnum<file>)  [unwired: 1 in, 2 out]
        n1726 = Read from Binary File(5:0.0, 8:w2703, 9:w2679, 10:w2680, 11:w2707) -> (0:w2702:errorcluster, 2:w2700:dbl[], 3:w2705:refnum<file>)  [unwired: 2 out]
        n1727 = Array To Cluster(array=w2700) -> (cluster=w2699:T56)
        n1728 = Unbundle(w2699) -> ("[0]"=w2667:dbl, "[1]"=w2665:dbl, "[2]"=w2666:dbl, "[3]"=w2664:dbl, "[4]"=w2698:dbl, "[5]"=w2697:dbl)
        n1729 = Close File(refnum=w2705, error in=w2702) -> (error out=→"Read cal error":errorcluster)  [unwired: 1 out]
        n1730 = Multiply(x=w2698, y=w2696) -> (x*y=w2693:dbl)
        n1731 = Multiply(x=w2697, y=w2696) -> (x*y=w2689:dbl)
        n1732 = Read from Binary File(5:0.0, 9:w2679, 10:w2680, 11:w2681) -> (2:w2675:dbl[], 3:w2673:refnum<file>)  [unwired: 1 in, 3 out]
        n1733 = Close File(refnum=w2673) -> ()  [unwired: 1 in, 2 out]
        n1734 = Bundle By Name(cluster="T1 calibration", "T1 alpha_x (nm/V)"=w2667, "T1 offset_x (mV)"=w2693, "T1 kappa_x (pN/nm)"=w2666) -> (w2692:T9)
        n1735 = Array Subset(array=w2675, index=1) -> (w2672:dbl[])  [unwired: 1 in]
        n1736 = Bundle By Name(cluster="T2 calibration", "T2 alpha_x (nm/V)"=w2665, "T2 offset_x (mV)"=w2689, "T2 kappa_x (pN/nm)"=w2664) -> (w2690:T8)
        n1737 = Index Array(array=w2675, index=0) -> (element=→"Offset file step size":dbl)
        n1738 = local write "T1 calibration"(w2692) -> ()
        n1739 = local write "T2 calibration"(w2690) -> ()
        n1740 = Decimate 1D Array(w2672) -> (w2662:dbl[], w2661:dbl[])  [unwired: 1 out]
        n1741 = Multiply(x=w2667, y=w2666) -> (x*y=w2668:dbl)
        n1742 = Multiply(x=w2665, y=w2664) -> (x*y=w2669:dbl)
        n1743 = Divide(x=w2669, y=w2668) -> (x/y=w2660:dbl)
        n1744 = property on="B factor" class="DigNum (strict)"("Val(Sgnl)"=w2660) -> ()  [unwired: 2 in, 2 out]
        n1745 = Bundle By Name(cluster="Offset Values", "Trap 1X offset"=w2662, "Trap 2X offset"=w2661) -> (w2670:T20)
        n1746 = Multiply(x=w2661, y=w2660) -> (x*y=w2663:dbl[])
        n1747 = local write "Offset Values"(w2670) -> ()
        n1748 = Subtract(x=w2662, y=w2663) -> (x-y=w2658:dbl[])
        n1749 = case shown="True" "Auto read offset correction" {
          tunnel: w2658 -> [_ w2716]
          frame False {
          }
          frame True {
            n1750 = property on="Setpoint offset\ncorrection values" class="Arr (strict)"("Val(Sgnl)"=w2716) -> ()  [unwired: 2 in, 2 out]
          }
        }
      }
      event "Abort MCL Scan": Value Change {
        n1751 = event-data() -> ()  [unwired: 7 out]
        n1752 = local write "MCL Scanning"(FALSE ("MCL Scanning")) -> ()
        n1753 = xnode "Read/Write Control"("FPGA VI Reference In"=w2717, "Abort scan (MCL)"="Abort MCL Scan") -> ("error out"=w2720:errorcluster)  [unwired: 1 in, 1 out]
      }
      event "Update Count (MCL)": Value Change {
        n1754 = event-data() -> ()  [unwired: 7 out]
        n1755 = xnode "Read/Write Control"("FPGA VI Reference In"=w2721, "MCL count"="Update Count (MCL)") -> ("error out"=w2723:errorcluster)  [unwired: 1 in, 1 out]
      }
      event "+ phase (MCL)", "- phase (MCL)": Value Change {
        n1756 = event-data() -> ()  [unwired: 7 out]
        n1757 = Or(x="- phase (MCL)", y="+ phase (MCL)") -> (x .or. y?=w2727:bool)
        n1758 = Negate(x="Phase adjust (MCL)") -> (-x=w2733:i16)
        n1759 = Select(t=w2733, s="+ phase (MCL)", f="Phase adjust (MCL)") -> (s? t:f=w2731:i16)
        n1760 = xnode "Read/Write Control"("FPGA VI Reference In"=w2724, "Phase count adjustment (MCL)"=w2731) -> ("FPGA VI Reference Out"=w2728:T50, "error out"=w2729:errorcluster)  [unwired: 1 in]
        n1761 = xnode "Read/Write Control"("FPGA VI Reference In"=w2728, "error in"=w2729, "+ phase (MCL)"=w2727) -> ("error out"=w2726:errorcluster)  [unwired: 1 out]
      }
      event "Abort AOD Scan": Value Change {
        n1762 = event-data() -> ()  [unwired: 7 out]
        n1763 = xnode "Read/Write Control"("FPGA VI Reference In"=w2734, "Abort scan"="Abort AOD Scan") -> ("error out"=w2736:errorcluster)  [unwired: 1 in, 1 out]
      }
      event "Continuous AOD Scanning": Value Change {
        n1764 = event-data() -> ()  [unwired: 7 out]
        n1765 = xnode "Read/Write Control"("FPGA VI Reference In"=w2737, "Cont. Scan"="Continuous AOD Scanning") -> ("error out"=w2739:errorcluster)  [unwired: 1 in, 1 out]
      }
      event "Index": Value Change {
        n1766 = event-data() -> ()  [unwired: 7 out]
        n1767 = call "Create new save file.vi"("Insert"="", "Ext"=".dat" ("string"), "Index In"="Index") -> ("Path Out"=→"Save file name":path, "Index Out"=w2740:dbl)
        "Save index" <- w2740
        n1768 = local write "Index"(w2740) -> ()
      }
      event "AO1", "AO2": Value Change {
        w2754 = 10.0 ("y")
        w2753 = 32767.0 ("y")
        n1769 = event-data() -> ()  [unwired: 7 out]
        n1770 = local read "AO2"() -> (w2752:dbl)
        n1771 = local read "AO1"() -> (w2749:dbl)
        n1772 = Multiply(x=w2749, y=w2753) -> (x*y=w2748:dbl)
        n1773 = Multiply(x=w2752, y=w2753) -> (x*y=w2751:dbl)
        n1774 = Divide(x=w2748, y=w2754) -> (x/y=w2747:dbl)
        n1775 = Divide(x=w2751, y=w2754) -> (x/y=w2750:dbl)
        n1776 = To Word Integer(number=w2747) -> (16bit integer=w2755:i16)
        n1777 = To Word Integer(number=w2750) -> (16bit integer=w2756:i16)
        n1778 = xnode "Read/Write Control"("FPGA VI Reference In"=w2745, "AO1"=w2755, "AO2"=w2756) -> ("error out"=w2746:errorcluster)  [unwired: 1 in, 1 out]
      }
      event "Inject Pump 1": Value Change {
        n1779 = event-data() -> ()  [unwired: 7 out]
        n1780 = disable-structure shown="Disabled" {
          disable-tunnel: w2757 -> [w2758 _]
          frame Disabled {
            n1781 = local read "Use Harvard pumps\nfor beads (else Chemyx)"() -> (w2759:bool)
            n1782 = case shown="True" w2759 {
              tunnel: "Inject Pump 1" -> [w2763 w2804]
              tunnel: w2758 -> [_ w2805]
              frame False {
                n1783 = local read "Pump write delay (ms)"() -> (w2762:dbl)
                n1784 = local read "Chemyx Syringe Pump Serial Port"() -> (w2761:refnum<visa-resource-name>)
                n1785 = case shown="True" w2763 {
                  tunnel: w2762 -> [w2769 w2783]
                  tunnel: w2761 -> [w2766 w2782]
                  frame False {
                    n1786 = flat-sequence {
                      tunnel: w2766 -> [w2770]
                      tunnel: [w2770] -> w2767
                      tunnel: w2769 -> [_]
                      tunnel: [w2773] -> w2768
                      tunnel: w2767 -> [w2773]
                      tunnel: w2768 -> [w2774]
                      tunnel: [w2774] -> w2764
                      tunnel: [w2776] -> w2765
                      tunnel: w2764 -> [w2776]
                      tunnel: w2765 -> [w2778]
                      frame #0 {
                        n1787 = call "Write to pump.vi"("string"="enter pump1", "VISA resource name"=w2770) -> ()  [unwired: 1 out]
                      }
                      frame #1 {
                        n1788 = Wait (ms)(milliseconds to wait="Pump pause delay (ms)") -> ()  [unwired: 1 out]
                      }
                      frame #2 {
                        n1789 = call "Write to pump.vi"("string"="stop", "VISA resource name"=w2774) -> ()  [unwired: 1 out]
                      }
                      frame #3 {
                        n1790 = Wait (ms)(milliseconds to wait=u32 500) -> ()  [unwired: 1 out]
                      }
                      frame #4 {
                        n1791 = call "Write to pump.vi"("string"="stop", "VISA resource name"=w2778) -> ()  [unwired: 1 out]
                      }
                    }
                  }
                  frame True {
                    n1792 = flat-sequence {
                      tunnel: w2782 -> [w2792]
                      tunnel: w2783 -> [w2787]
                      tunnel: w2783 -> [w2794]
                      tunnel: w2782 -> [w2795]
                      tunnel: [w2795] -> w2780
                      tunnel: [w2797] -> w2781
                      tunnel: w2780 -> [w2797]
                      tunnel: w2781 -> [w2799]
                      frame #0 {
                        n1793 = local read "All Pump Parameters"() -> (w2786:T10)
                        n1794 = Unbundle By Name(w2786) -> ("Pump 1"=w2793:T57)
                        n1795 = call "Set pump parameters.vi"("Pump write delay (ms)"=w2787, "Volume (uL)"="Ch 1 Inject Volume (uL)", "Rate (uL/h)"="Ch 1 Inject Rate (ul/h)", "Units"=4.0, "Pump #"=1.0, "Pump Parameters In"=w2793, "VISA resource name"=w2792) -> ("Pump Parameters Out"=w2785:T57)  [unwired: 3 in]
                        n1796 = Bundle By Name(cluster=w2786, "Pump 1"=w2785) -> (w2784:T10)
                        n1797 = local write "All Pump Parameters"(w2784) -> ()
                      }
                      frame #1 {
                        n1798 = Wait (ms)(milliseconds to wait=w2794) -> ()  [unwired: 1 out]
                      }
                      frame #2 {
